vi "Append Image.vi"(1 "Cell Address":string, 4 "Image Path":path, 6 "error in (no error)":errorcluster, 7 "Column Index":i32, 8 "Caption":string, 9 "Row Index":i32, 10 "Report Ref In":T2) -> (0 "error out":errorcluster, 2 "Image Index":i32, 3 "Report Ref Out":T2)   [LabVIEW 2013, in "XCel Report Engine.lvlib"]
doc: "Inserts an image into the active worksheet and anchors it to a cell.\n\nThe insertion position can be specified using an Excel A1 cell address or zero-based row and column coordinates. When Cell Address is not empty, it takes precedence over the numeric coordinates. Coordinate (0, 0) corresponds to cell A1.\n\nThe image is embedded in the workbook and does not retain an external link to the source file. Repeated insertion of the same image data within a worksheet reuses the embedded media when possible.\n\nPicture Index returns the zero-based index of the inserted image and can be passed to Format Image.vi.\n\nAlignment and Caption are retained for compatibility with the NI Report Generation Toolkit. They do not affect image placement or content in Excel reports."
uses:
  XCel Report Engine.lvlib
  C:/Users/m.santucci/Documents/ChatGPT/LV_REPORT_ENGINE/LV/DotNet/XCelReportEngine.dll
  LV/DotNet/XCelReportEngine.dll
  Controls/Report Ref.ctl
  Controls/Image Alignment.ctl
panel:
  in  "Image Alignment":T1
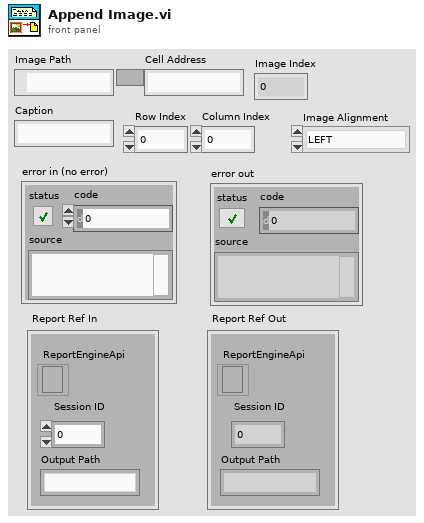
[diagram p1: front panel]
types:
  T1 = typedef "XCel Report Engine.lvlib/Image Alignment.ctl" = enum32{"LEFT", "RIGHT", "TOP", "TEXTTOP", "MIDDLE", "ABSMIDDLE", "BASELINE", "BOTTOM", "ABSBOTTOM"}
  T2 = typedef "XCel Report Engine.lvlib/Report Ref.ctl" = cluster{"Session ID":i32, "Output Path":string, "ReportEngineApi":refnum<k24>}
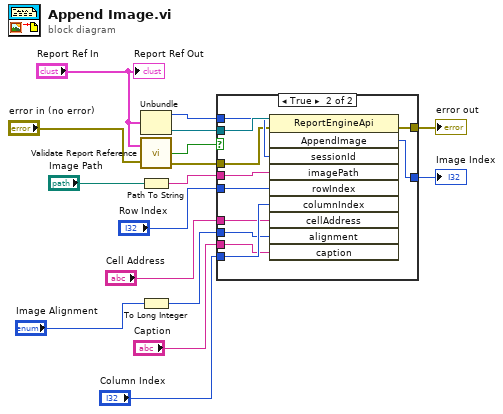
[diagram p0: block diagram]
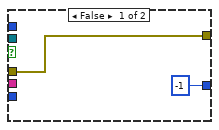
[diagram p2: hidden frame]
diagram:
  n1 = Unbundle("Report Ref In") -> ("Session ID"=w14:i32, "ReportEngineApi"=w16:refnum<k24>)  [unwired: 1 out]
  n2 = call "Validate Report Reference.vi"("Report Ref In"="Report Ref In", "error in (no error)"="error in (no error)") -> ("Valid"=w1:bool, "error out"=w2:errorcluster)  [unwired: 1 out]
  n3 = Path To String(path="Image Path") -> (string=w10:string)
  n4 = To Long Integer(number="Image Alignment") -> (32bit integer=w6:i32)
  n5 = case shown="True" w1 {
    tunnel: w16 -> [_ w29]
    tunnel: [w18 w28] -> w15
    tunnel: w14 -> [_ w27]
    tunnel: "Row Index" -> [_ w26]
    tunnel: "Column Index" -> [_ w25]
    tunnel: w10 -> [_ w24]
    tunnel: "Caption" -> [_ w23]
    tunnel: "Cell Address" -> [_ w22]
    tunnel: [-1 ("AppendImage") w21] -> w7
    tunnel: w6 -> [_ w20]
    tunnel: w2 -> [w18 w19]
    frame False {
    }
    frame True {
      n6 = invoke class="ReportEngineApi" method="AppendImage"(reference=w29, error in=w19, "sessionId"=w27, "imagePath"=w24, "rowIndex"=w26, "columnIndex"=w25, "cellAddress"=w22, "alignment"=w20, "caption"=w23) -> (error out=w28:errorcluster, "AppendImage"=w21:i32)  [unwired: 1 in, 8 out]
    }
  }
  "error out" <- w15
  "Image Index" <- w7
  "Report Ref Out" <- "Report Ref In"
